vi "Configure.vi"(8 "error in (no error)":errorcluster, 9 "Record":bool=TRUE, 10 "Recording Channels":refnum<k21>="State System Analog Input", 11 "BehaviorData in":refnum<class "BehaviorData.lvclass">) -> (0 "error out":errorcluster, 3 "BehaviorData out":refnum<class "BehaviorData.lvclass">)   [LabVIEW 2014, in "BehaviorData.lvclass"]
uses:
  BehaviorData.lvclass
  BehaviorData.lvclass/BehaviorData.ctl
  <vilib>/DAQmx/create/channels.llb/DAQmx Create Channel (CI-Count Edges).vi
  AcquireTraces/AcquireTraces.lvclass
  <resource>/objmgr/daqmx.rc
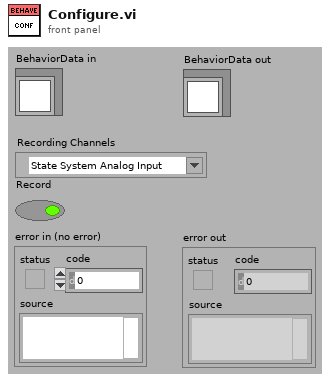
[diagram p1: front panel]
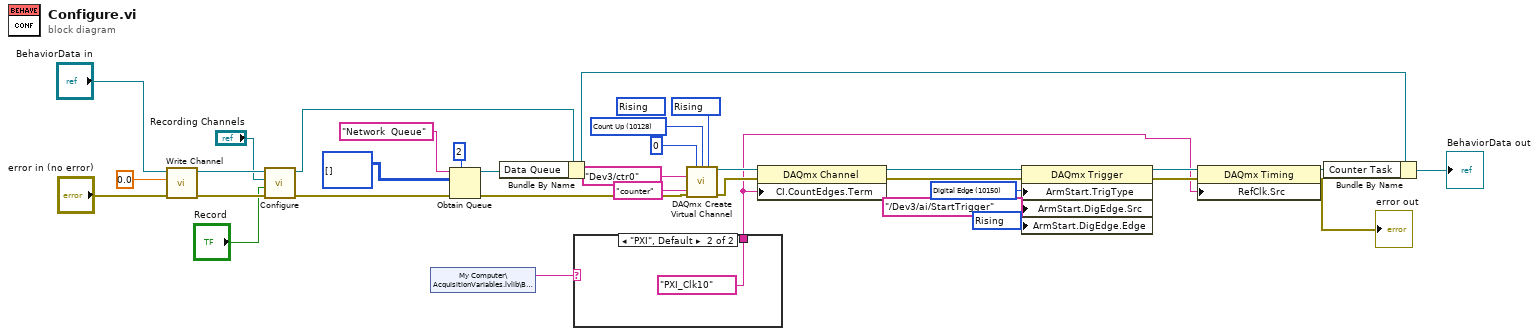
[diagram p0: block diagram]
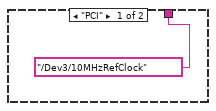
[diagram p2: hidden frame]
diagram:
  w11 = 10280 items=["Rising"=10280, "Falling"=10171] ("edge")
  w15 = 10280 items=["Rising"=10280, "Falling"=10171] ("ArmStart.DigEdge.Edge")
  w17 = 10150 items=["Digital Edge"=10150, "None"=10230] ("ArmStart.TrigType")
  (unwired) 10280 items=["Rising"=10280, "Falling"=10171] ("edge")
  w22 = 10128 items=["Count Up"=10128, "Count Down"=10124, "Externally Controlled"=10326] ("count direction")
  n1 = call-dynamic "Write Channel.vi"("error in (no error)"="error in (no error)", "Channel"=0.0, "AcquistionObject in"="BehaviorData in") -> ("error out"=w30:errorcluster, "AcquistionObject out"=w32:refnum<class "BehaviorData.lvclass">)  [unwired: 7 in]
  n2 = call-parent "Configure.vi"("error in (no error)"=w30, "Record"="Record", "Recording Channels"="Recording Channels", "AcquireTraces in"=w32) -> ("error out"=w25:errorcluster, "AcquireTraces out"=w27:refnum<class "BehaviorData.lvclass">)  [unwired: 6 in]
  n3 = shared-variable "My Computer\\AcquisitionVariables.lvlib\\Bus System"() -> (w2:string)  [unwired: 1 in, 1 out]
  n4 = Obtain Queue(max queue size (-1, unlimited)=2, name (unnamed)="Network  Queue", element data type=i32[][] [], error in (no error)=w25) -> (queue out=w26:refnum<queue>, error out=w12:errorcluster)  [unwired: 1 in, 1 out]
  n5 = Bundle By Name(cluster=w27, "Data Queue"=w26) -> (w14:refnum<class "BehaviorData.lvclass">)
  n6 = case shown="\"PXI\", Default" w2 {
    tunnel: [tag "/Dev3/10MHzRefClock" ("CI.CountEdges.Term") tag "PXI_Clk10" ("CI.CountEdges.Term")] -> w1
    frame "PCI" {
    }
    frame "PXI", Default {
    }
  }
  n7 = call-poly <vilib>:"DAQmx Create Virtual Channel.vi"("initial count"=u32 0, "count direction"=w22, "edge"=w11, "counter"=tag "Dev3/ctr0", "name to assign"="counter", "error in"=w12) -> ("task out"=w20:refnum<k21>, "error out"=w19:errorcluster)  [unwired: 8 in]
  n8 = property class="DAQmx Channel"(reference=w20, error in=w19, "CI.CountEdges.Term"=w1) -> (reference out=w18:refnum<k21>, error out=w13:errorcluster)
  n9 = property class="DAQmx Trigger"(reference=w18, error in=w13, "ArmStart.TrigType"=w17, "ArmStart.DigEdge.Src"=tag "/Dev3/ai/StartTrigger", "ArmStart.DigEdge.Edge"=w15) -> (reference out=w6:refnum<k21>, error out=w4:errorcluster)
  n10 = property class="DAQmx Timing"(reference=w6, error in=w4, "RefClk.Src"=w1) -> (reference out=w5:refnum<k21>, error out=→"error out":errorcluster)
  n11 = Bundle By Name(cluster=w14, "Counter Task"=w5) -> (→"BehaviorData out":refnum<class "BehaviorData.lvclass">)
